vi "Lecutra_DB_log.vi"(11 "HMI Class 3.lvclass":refnum<class "HMI Class 3.lvclass">) -> (3 "HMI Class 3.lvclass 2":refnum<class "HMI Class 3.lvclass">)   [LabVIEW 2019, in "HMI Class 3.lvclass"]
uses:
  HMI Class 3.lvclass
  HMI Class 3.lvclass/HMI Class 3.ctl
  <vilib>/addons/database/Connection.llb/DB Tools Open Connec (Path).vi
  <vilib>/addons/database/_DB Variant To Data/Database Variant To Data.xnode
  <vilib>/addons/database/NI_Database_API.lvlib
panel:
  out "error out":errorcluster
  in  "error in (no error)":errorcluster
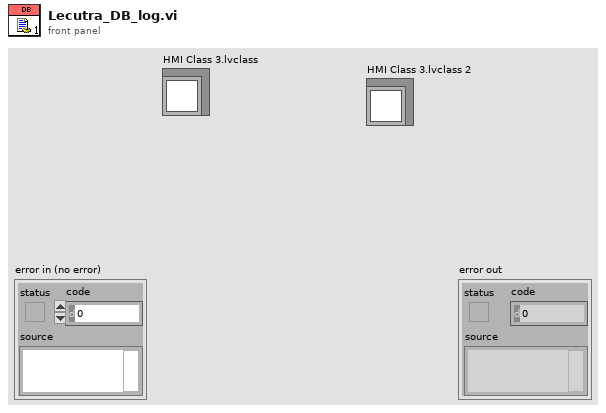
[diagram p1: front panel]
types:
  T1 = typedef "NI_Database_API.lvlib/Conn ObjectReference.ctl" = refnum<k1>
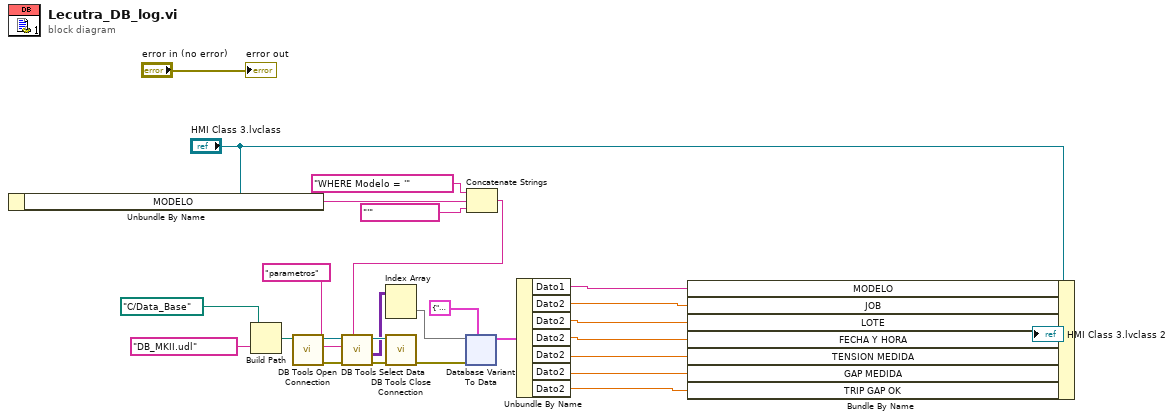
[diagram p0: block diagram]
diagram:
  n1 = Unbundle By Name("HMI Class 3.lvclass") -> ("MODELO"=w10:string)
  n2 = Build Path(base path=path "C:/Data_Base", name or relative path="DB_MKII.udl") -> (appended path=w18:path)
  n3 = call-poly <vilib>:"DB Tools Open Connection.vi"("connection information"=w18) -> ("error out"=w21:errorcluster, "connection reference"=w20:T1)  [unwired: 7 in]
  n4 = Concatenate Strings("WHERE Modelo = '" ("string"), w10, "'" ("string")) -> (w8:string)
  n5 = call <vilib>:"DB Tools Select Data.vi"("condition"=w8, "error in (no error)"=w21, "table"="parametros", "connection reference"=w20) -> ("error out"=w25:errorcluster, "data"=w23:variant[][], "connection reference out"=w24:T1)  [unwired: 2 in]
  n6 = Index Array(array=w23) -> (element=w22:variant[])  [unwired: 2 in]
  n7 = call <vilib>:"DB Tools Close Connection.vi"("error in (no error)"=w25, "connection reference"=w24) -> ("error out"=w17:errorcluster)  [unwired: 5 in]
  n8 = xnode "Database Variant To Data"("database variant"=w22, "error in (no error)"=w17, "type"=cluster{"Dato1":string, "Dato2":dbl} {"Dato1"="", "Dato2"=0.0} ("Parametros")) -> ("data"=w15:cluster{"Dato1":string, "Dato2":dbl})  [unwired: 1 out]
  n9 = Unbundle By Name(w15) -> ("Dato1"=w12:string, "Dato2"=w6:dbl, "Dato2"=w5:dbl, "Dato2"=w4:dbl, "Dato2"=w3:dbl, "Dato2"=w2:dbl, "Dato2"=w1:dbl)
  n10 = Bundle By Name(cluster="HMI Class 3.lvclass", "MODELO"=w12, "JOB"=w6, "LOTE"=w5, "FECHA Y HORA"=w4, "TENSION MEDIDA"=w3, "GAP MEDIDA"=w2, "TRIP GAP OK"=w1) -> (→"HMI Class 3.lvclass 2":refnum<class "HMI Class 3.lvclass">)
  "error out" <- "error in (no error)"
